vi "Get Mouse Pos LAT LONG.vi"(8 "error in (no error)":errorcluster, 11 "GMapControl reference":refnum<k24>) -> (0 "error out":errorcluster, 1 "FromLocalToLatLng":refnum<k24>, 2 "Lng":dbl, 3 "Lat":dbl, 5 "Y":i32, 7 "X":i32)   [LabVIEW 2014]
uses:
  C:/Robotic Systems/Products/Surveyor/Software/Ground Station/Data/Mapping DLL/GMap.NET.WindowsForms.dll
  Data/Mapping DLL/GMap.NET.WindowsForms.dll
  C:/Robotic Systems/Products/Surveyor/Software/Ground Station/Data/Mapping DLL/GMap.NET.Core.dll
  Data/Mapping DLL/GMap.NET.Core.dll
  System.Windows.Forms
  System.Drawing
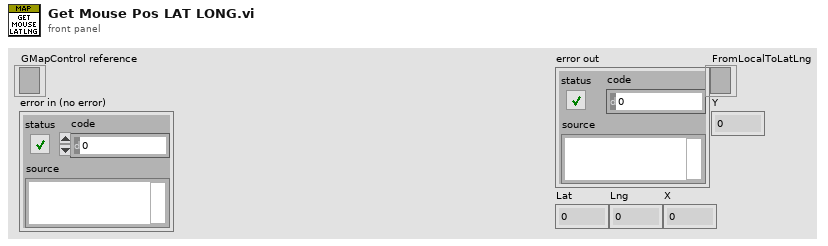
[diagram p1: front panel]
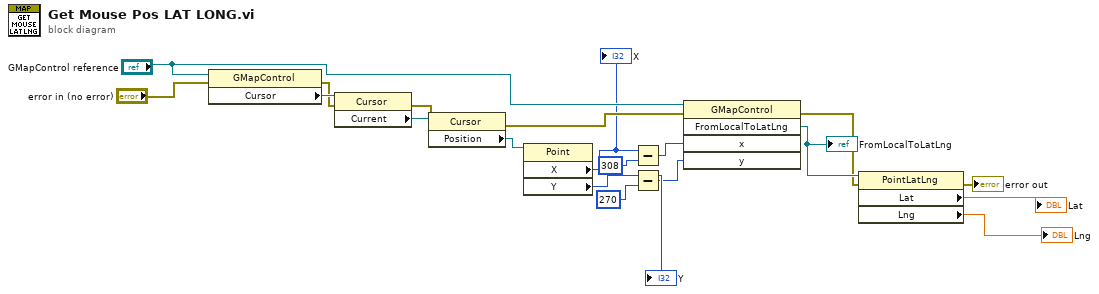
[diagram p0: block diagram]
diagram:
  n1 = property class="GMapControl"(reference="GMapControl reference", error in="error in (no error)") -> (error out=w16:errorcluster, "Cursor"=w19:refnum<k24>)  [unwired: 1 out]
  n2 = property class="Cursor"(reference=w19, error in=w16) -> (error out=w15:errorcluster, "Current"=w18:refnum<k24>)  [unwired: 1 out]
  n3 = property class="Cursor"(reference=w18, error in=w15) -> (error out=w14:errorcluster, "Position"=w8:refnum<k24>)  [unwired: 1 out]
  n4 = property class="Point"(reference=w8) -> ("X"=w4:i32, "Y"=w6:i32)  [unwired: 1 in, 2 out]
  "X" <- w4
  "Y" <- w6
  n5 = Subtract(x=w4, y=308) -> (x-y=w2:i32)
  n6 = Subtract(x=w6, y=270) -> (x-y=w1:i32)
  n7 = invoke class="GMapControl" method="FromLocalToLatLng"(reference="GMapControl reference", error in=w14, "x"=w2, "y"=w1) -> (error out=w13:errorcluster, "FromLocalToLatLng"=w17:refnum<k24>)  [unwired: 1 in, 3 out]
  "FromLocalToLatLng" <- w17
  n8 = property class="PointLatLng"(reference=w17, error in=w13) -> (error out=→"error out":errorcluster, "Lat"=→"Lat":dbl, "Lng"=→"Lng":dbl)  [unwired: 1 out]
